vi "RxCALON.vi"(4 "PhyPort":u32, 6 "WaveformName(WithType)":string, 7 "VISAName":string="TCPIP0::10.144.41.48::inst0::INSTR", 8 "PacketNumber":i32, 9 "RxPwr":dbl, 10 "Freq(Hz)":dbl, 11 "ExternalAtt":dbl) -> ()   [LabVIEW 2015]
uses:
  VISAOperation.ctl
  ONOFF.ctl
  PhyPort.ctl
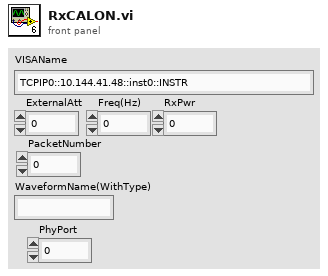
[diagram p1: front panel]
types:
  T1 = typedef "PhyPort.ctl" = enum16{"Port0", "Port1", "Port2", "Port3", "Port4", "Port5", "Port6", "Port7"}
  T2 = cluster{"ExternalAtt":dbl, "Freq":dbl, "RxPwr":dbl, "PacketNumber":i32, "WaveformName(WithType)":string, "PhyPort":T1}
  T3 = typedef "ONOFF.ctl" = u16
  T4 = typedef "VISAOperation.ctl" = enum16{"RunFile", "OpenDebugPanel", "ReadError", "ReadSTB", "Reset", "Clean", "CloseVISA", "RunCMD", "OpenVISA"}
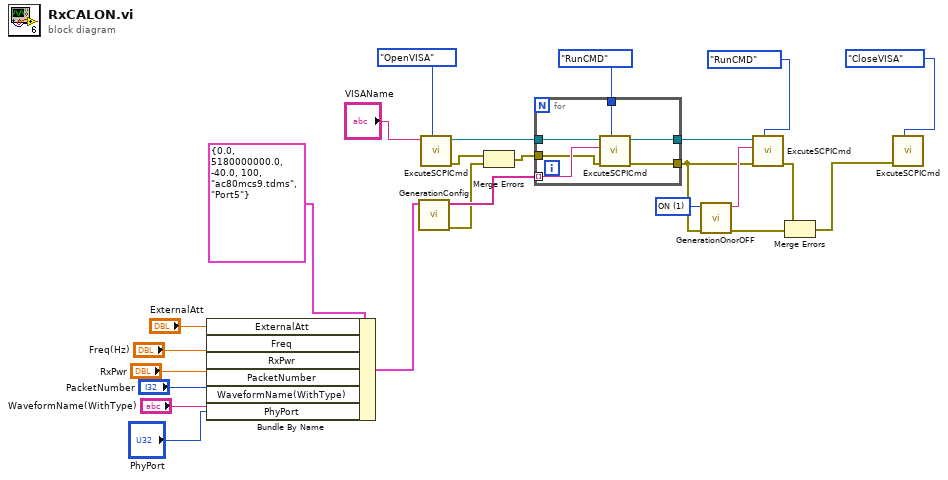
[diagram p0: block diagram]
diagram:
  w11 = T3 1 items=["OFF", "ON"] ("ON/OFF")
  n1 = Bundle By Name(cluster=T2 {"ExternalAtt"=0.0, "Freq"=5180000000.0, "RxPwr"=-40.0, "PacketNumber"=100, "WaveformName(WithType)"="ac80mcs9.tdms", "PhyPort"=enum."Port5"} ("GenerationConfig"), "ExternalAtt"="ExternalAtt", "Freq"="Freq(Hz)", "RxPwr"="RxPwr", "PacketNumber"="PacketNumber", "WaveformName(WithType)"="WaveformName(WithType)", "PhyPort"="PhyPort") -> (w3:T2)
  n2 = call "GenerationConfig.vi"("GenerationConfig"=w3) -> ("error out"=w16:errorcluster, "GenerationConfigCMD"=w22:string[])  [unwired: 9 in]
  n3 = call "ExcuteSCPICmd.vi"("VISAOperation"=VISAOperation."OpenVISA", "VISA resource name"="VISAName") -> ("error out"=w17:errorcluster, "reference out"=w24:refnum<visa-resource-name>)  [unwired: 6 in, 2 out]
  n4 = Merge Errors(w17, w16) -> (w15:errorcluster)
  n5 = for {
    tunnel: w24 -> [w31]
    tunnel: VISAOperation."RunCMD" ("VISAOperation") -> [w30]
    tunnel: w22 -> [w29] mode=indexing
    tunnel: [w28] -> w21
    tunnel: w15 -> [w27]
    tunnel: [w26] -> w14
    n6 = call "ExcuteSCPICmd.vi"("VISAOperation"=w30, "error in (no error)"=w27, "Run Command"=w29, "VISA resource name"=w31) -> ("error out"=w26:errorcluster, "reference out"=w28:refnum<visa-resource-name>)  [unwired: 4 in, 2 out]
  }
  n7 = call "GenerationOnorOFF.vi"("error in (no error)"=w14, "ON/OFF"=w11) -> ("error out"=w13:errorcluster, "ON/OFFCMD"=w19:string)  [unwired: 8 in]
  n8 = call "ExcuteSCPICmd.vi"("VISAOperation"=VISAOperation."RunCMD", "error in (no error)"=w14, "Run Command"=w19, "VISA resource name"=w21) -> ("error out"=w12:errorcluster)  [unwired: 4 in, 3 out]
  n9 = Merge Errors(w12, w13) -> (w10:errorcluster)
  n10 = call "ExcuteSCPICmd.vi"("VISAOperation"=VISAOperation."CloseVISA", "error in (no error)"=w10) -> ()  [unwired: 6 in, 4 out]
